vi "BuildCall.vi"(7 "PythonConverter_BD in":refnum<class "PyConvBD.lvclass">, 8 "error in":errorcluster, 11 "CaseStructure in":refnum<class "CaseStructure.lvclass">) -> (0 "error out":errorcluster, 3 "CaseStructure out":refnum<class "CaseStructure.lvclass">, 5 "PythonConverter_BD out":refnum<class "PyConvBD.lvclass">)   [LabVIEW 2014, in "CaseStructure.lvclass"]
uses:
  CaseStructure.lvclass
  Python/PythonConverter_BD/PyConvBD.lvclass
  Python/Parsing/ListTypesTD.ctl
  Python/PythonConverter_BD/TypeDefs/NodeCall_TD.ctl
  Tunnel/Tunnel.lvclass
  Python/Parsing/Python Functions.lvlib
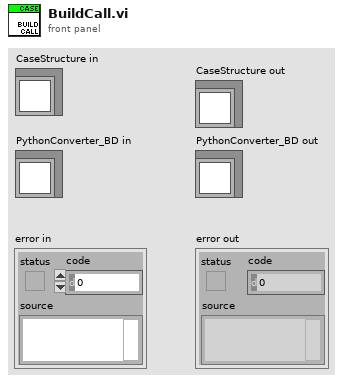
[diagram p1: front panel]
types:
  T1 = typedef "NodeCall_TD.ctl" = cluster{"call":string, "collect":string, "Threaded":bool, "branches":string[]}
  T2 = typedef "Python Functions.lvlib/ListTypesTD.ctl" = enum16{"list", "tuple", "parameter list", "output list"}
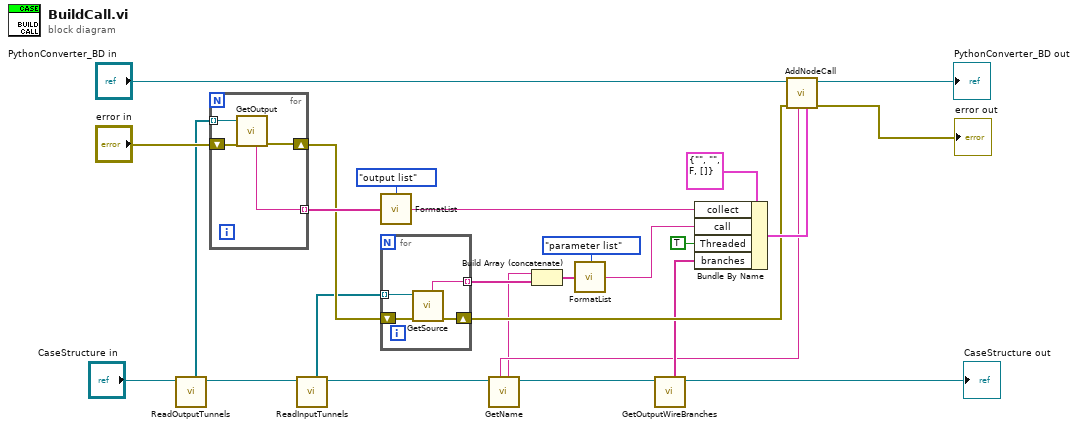
[diagram p0: block diagram]
diagram:
  n1 = call-dynamic "ReadOutputTunnels.vi"("Structure in"="CaseStructure in") -> ("Structure out"=w17:refnum<class "CaseStructure.lvclass">, "outputs"=w18:refnum<class "Tunnel.lvclass">[])  [unwired: 7 in]
  n2 = for {
    tunnel: w18 -> [w30] mode=indexing
    shift-right: [w27] -> w16
    shift-left: "error in" -> [w29]
    tunnel: [w28] -> w24 mode=indexing
    n3 = call-dynamic "GetOutput.vi"("error in"=w29, "Tunnel in"=w30) -> ("error out"=w27:errorcluster, "name"=w28:string)  [unwired: 5 in, 1 out]
  }
  n4 = call-dynamic "ReadInputTunnels.vi"("Structure in"=w17) -> ("Structure out"=w4:refnum<class "CaseStructure.lvclass">, "tunnels"=w15:refnum<class "Tunnel.lvclass">[])  [unwired: 7 in]
  n5 = call "FormatList.vi"("values"=w24, "type"=ListTypesTD."output list") -> ("python object"=w13:string)
  n6 = for {
    tunnel: w15 -> [w34] mode=indexing
    shift-right: [w32] -> w9
    shift-left: w16 -> [w33]
    tunnel: [w31] -> w11 mode=indexing
    n7 = call-dynamic "GetSource.vi"("error in"=w33, "Tunnel in"=w34) -> ("error out"=w32:errorcluster, "name"=w31:string)  [unwired: 5 in, 1 out]
  }
  n8 = call-dynamic "GetName.vi"("CaseStructure in"=w4) -> ("CaseStructure out"=w3:refnum<class "CaseStructure.lvclass">, "name"=w1:string, "UID"=w2:string)  [unwired: 5 in, 1 out]
  n9 = Build Array (concatenate)(w1, w11) -> (w10:string[])
  n10 = call "FormatList.vi"("values"=w10, "type"=ListTypesTD."parameter list") -> ("python object"=w8:string)
  n11 = call-dynamic "GetOutputWireBranches.vi"("CaseStructure in"=w3) -> ("CaseStructure out"=→"CaseStructure out":refnum<class "CaseStructure.lvclass">, "branches"=w5:string[])  [unwired: 6 in, 1 out]
  n12 = Bundle By Name(cluster=T1 {"call"="", "collect"="", "Threaded"=FALSE, "branches"=[]} ("call"), "collect"=w13, "call"=w8, "Threaded"=TRUE, "branches"=w5) -> (w12:T1)
  n13 = call "AddNodeCall.vi"("call"=w12, "name"=w2, "error in"=w9, "PythonConverter_BD in"="PythonConverter_BD in") -> ("error out"=→"error out":errorcluster, "PythonConverter_BD out"=→"PythonConverter_BD out":refnum<class "PyConvBD.lvclass">)  [unwired: 4 in]
